vi "Negate Formula String.vi"(2 "formula":string) -> (7 "- formula":string)   [LabVIEW 2021, in "Formula.lvlib"]
uses:
  Formula.lvlib
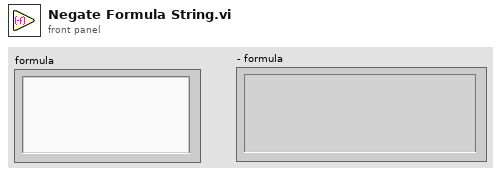
[diagram p1: front panel]
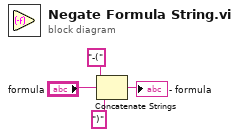
[diagram p0: block diagram]
diagram:
  n1 = Concatenate Strings("-(" ("string"), "formula", ")" ("string")) -> (→"- formula":string)
